vi "Get All Data Names.vi"(8 "error in (no error)":errorcluster, 11 "Json Data Reader in":refnum<class "Json Data Reader.lvclass">) -> (0 "error out":errorcluster, 2 "Data Names":string[](array[string]), 3 "Json Data Reader out":refnum<class "Json Data Reader.lvclass">)   [LabVIEW 2017, in "Json Data Reader.lvclass"]
uses:
  Json Data Reader.lvclass
  Json Data Reader.lvclass/Json Data Reader.ctl
  07f20b01-b216-4611-a5ec-fc74c5b156d0.vi
  <vilib>/JDP Science/JSONtext/Find Multiple Items.vi
  <vilib>/JDP Science/JSONtext/String Subset.vi
  <vilib>/JDP Science/JSONtext/support/Strip Quotes and Unescape.vi
  <vilib>/JDP Science/JSONtext/support/Unescape JSON string.vi
  <vilib>/JDP Science/JSONtext/Parsing/Parse Full Path or Item Name.vi
  <vilib>/JDP Science/JSONtext/Offset/Find Item Locations by Path.vi
  <vilib>/JDP Science/JSONtext/JSON text to Variant.vi
  <vilib>/JDP Science/JSONtext/LVClass Serializer/JSONtext LVClass Serializer.lvclass
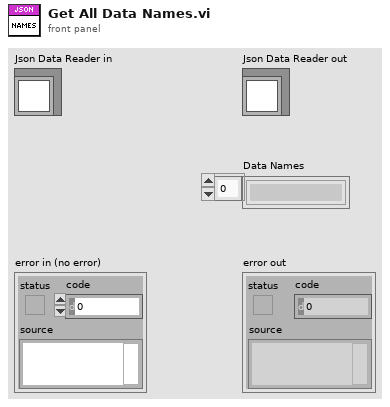
[diagram p1: front panel]
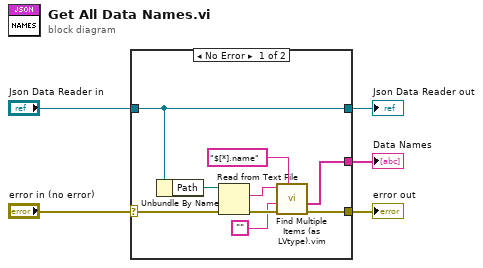
[diagram p0: block diagram]
diagram:
  n1 = case shown="No Error" "error in (no error)" {
    selector: "error in (no error)" -> [w14 w16]
    tunnel: [w10 w16] -> w4
    tunnel: [w12 w15] -> w2
    tunnel: "Json Data Reader in" -> [w12 w15]
    tunnel: [w6 _] -> w1
    frame No Error {
      n2 = Unbundle By Name(w12) -> ("Path"=w11:path)
      n3 = Read from Text File(file (use dialog)=w11, error in=w14) -> (text=w9:string, error out=w13:errorcluster)  [unwired: 2 in, 2 out]
      n4 = call "Find Multiple Items (as LVtype).vim"("$Path or Item Name"="$[*].name", "error in (no error)"=w13, "Data Type and Default Value"="", "JSON"=w9) -> ("error out"=w10:errorcluster, "Array of Data"=w6:string[])  [unwired: 4 in, 2 out]
    }
    frame Error {
    }
  }
  "error out" <- w4
  "Json Data Reader out" <- w2
  "Data Names" <- w1
